vi "get_increment.vi"(8 "error in (no error)":errorcluster, 11 "ImageCollection in":refnum<class "ImageCollection.lvclass">) -> (0 "error out":errorcluster, 1 "z increment":dbl[unit], 2 "time increment":dbl[unit], 3 "ImageCollection out":refnum<class "ImageCollection.lvclass">, 4 "type":T1)   [LabVIEW 2010, in "ImageCollection.lvclass"]
uses:
  ImageCollection.lvclass
  type_enum.ctl
  ImageCollection.lvclass/ImageCollection.ctl
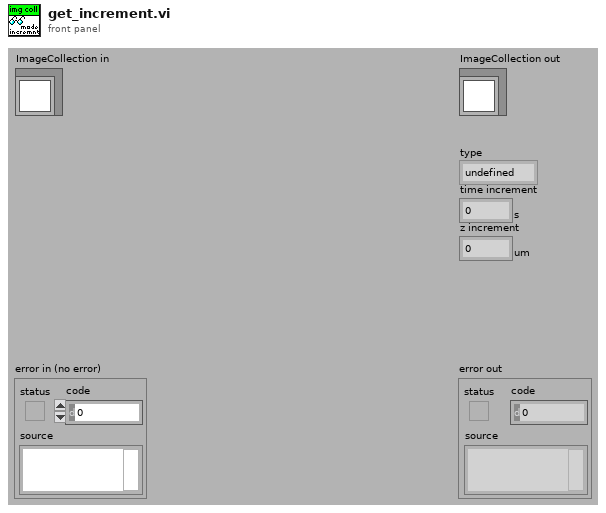
[diagram p1: front panel]
types:
  T1 = typedef "type_enum.ctl" = enum16{"undefined", "movie", "z-stack"}
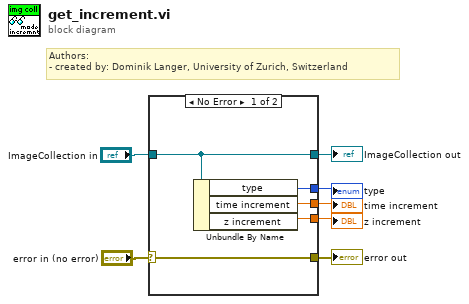
[diagram p0: block diagram]
diagram:
  # "Authors: \n- created by: Dominik Langer, University of Zurich, Switzerland"
  n1 = case shown="No Error" "error in (no error)" {
    selector: "error in (no error)" -> [w12 w14]
    tunnel: [w12 w14] -> w6
    tunnel: [w11 w13] -> w4
    tunnel: "ImageCollection in" -> [w11 w13]
    tunnel: [w10 _] -> w3
    tunnel: [w9 _] -> w2
    tunnel: [w8 _] -> w1
    frame No Error {
      n2 = Unbundle By Name(w11) -> ("type"=w10:T1, "time increment"=w9:dbl[unit], "z increment"=w8:dbl[unit])
    }
    frame Error {
    }
  }
  "error out" <- w6
  "ImageCollection out" <- w4
  "type" <- w3
  "time increment" <- w2
  "z increment" <- w1
